vi "Read dotNET Product Definitions.vi"(8 "error in (no error)":errorcluster, 10 "Product Definitions":refnum<k24>[](array[refnum]), 11 "Bundle Builder in":refnum<class "Bundle Builder.lvclass">) -> (0 "error out":errorcluster, 3 "Bundle Builder out":refnum<class "Bundle Builder.lvclass">)   [LabVIEW 2020, in "Bundle Builder.lvclass"]
uses:
  Bundle Builder.lvclass
  C:/Users/chihong/Documents/Repos/StsCustomBundleBuilder/Code/StsCustomBundleBuilderLib/StsCustomBundleBuilderLib/bin/Debug/StsCustomBundleBuilderLib.dll
  StsCustomBundleBuilderLib/StsCustomBundleBuilderLib/bin/Debug/StsCustomBundleBuilderLib.dll
  Bundle Builder.lvclass/Bundle Builder.ctl
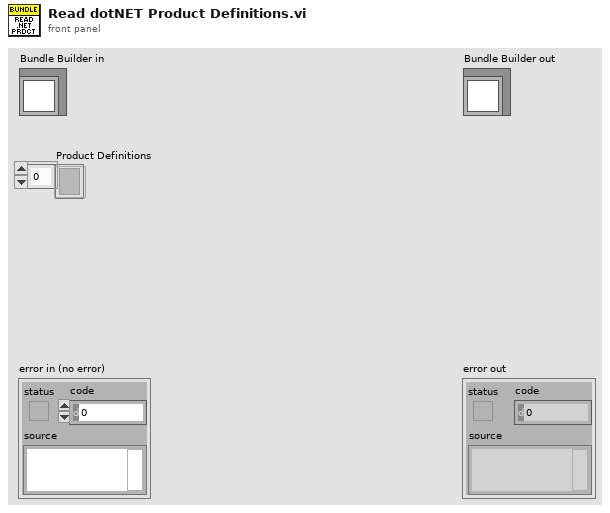
[diagram p1: front panel]
types:
  T1 = cluster{"Display Name":string, "Type":enum16{"NI Installer", "Custom Installer"}, "Install Commands":cluster{"Path":string, "Parameters":string, "Successful Exit Codes":string, "Log Command":cluster{"Flag":string, "File Name":string}}[], "Uninstall Commands":cluster{"Path":string, "Parameters":string, "Successful Exit Codes":string, "Log Command":cluster{"Flag":string, "File Name":string}}[]}
  T2 = cluster{"Path":string, "Parameters":string, "Successful Exit Codes":string, "Log Command":cluster{"Flag":string, "File Name":string}}
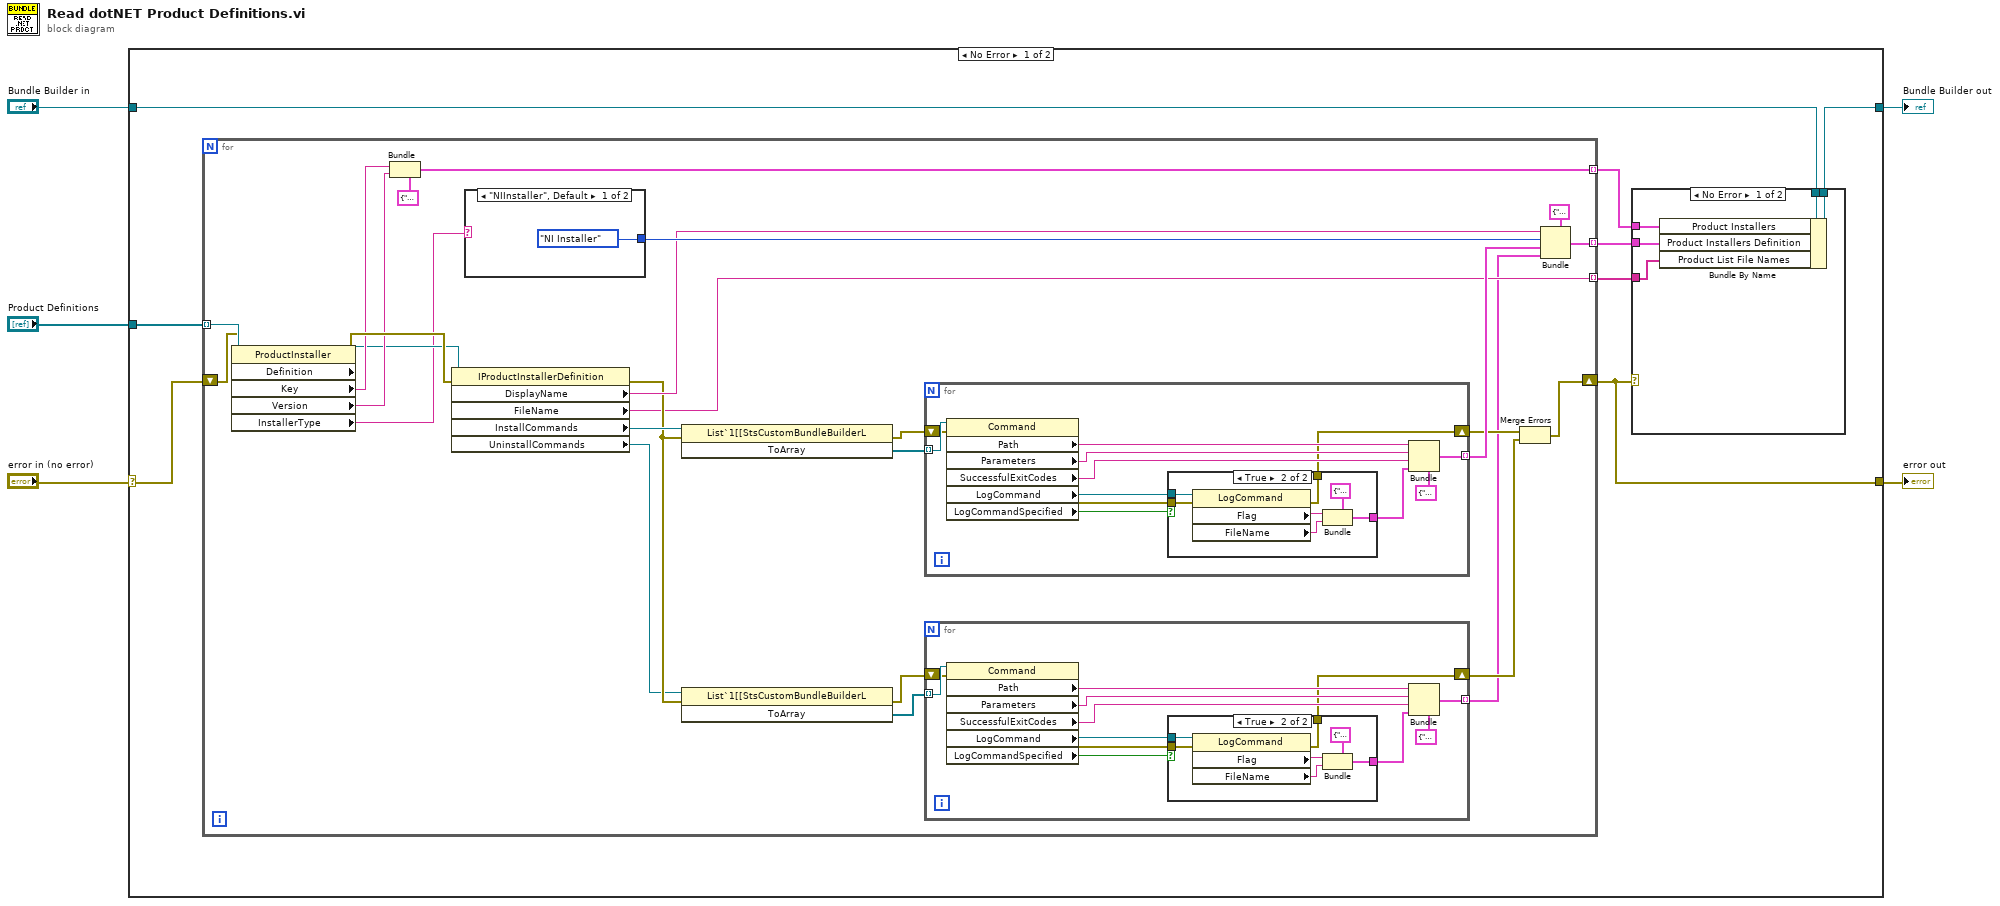
[diagram p0: block diagram]
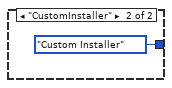
[diagram p5: hidden frame]
diagram:
  n1 = case shown="No Error" "error in (no error)" {
    selector: "error in (no error)" -> [w11 w89]
    tunnel: [w7 w89] -> w4
    tunnel: [w10 w88] -> w2
    tunnel: "Bundle Builder in" -> [w13 w88]
    tunnel: "Product Definitions" -> [w12 _]
    frame No Error {
      n2 = for {
        tunnel: w12 -> [w45] mode=indexing
        shift-right: [w27] -> w7
        shift-left: w11 -> [w44]
        tunnel: [w26] -> w9 mode=indexing
        tunnel: [w25] -> w8 mode=indexing
        tunnel: [w24] -> w6 mode=indexing
        n3 = property class="ProductInstaller"(reference=w45, error in=w44) -> (error out=w43:errorcluster, "Definition"=w38:refnum<k24>, "Key"=w41:string, "Version"=w40:string, "InstallerType"=w37:string)  [unwired: 1 out]
        n4 = Bundle(cluster=cluster{"Key":string, "Version":string} {"Key"="", "Version"=""} ("Product Installer"), "Key"=w41, "Version"=w40) -> (w25:cluster{"Key":string, "Version":string})
        n5 = property class="IProductInstallerDefinition"(reference=w38, error in=w43) -> (error out=w33:errorcluster, "DisplayName"=w35:string, "FileName"=w24:string, "InstallCommands"=w34:refnum<k24>, "UninstallCommands"=w32:refnum<k24>)  [unwired: 1 out]
        n6 = case shown="\"NIInstaller\", Default" w37 {
          tunnel: [enum16{"NI Installer", "Custom Installer"}."NI Installer" ("Type") enum16{"NI Installer", "Custom Installer"}."Custom Installer" ("Type")] -> w36
          frame "NIInstaller", Default {
          }
          frame "CustomInstaller" {
          }
        }
        n7 = invoke class="List`1[[StsCustomBundleBuilderL" method="ToArray"(reference=w34, error in=w33) -> (error out=w30:errorcluster, "ToArray"=w31:refnum<k24>[])  [unwired: 1 in, 1 out]
        n8 = invoke class="List`1[[StsCustomBundleBuilderL" method="ToArray"(reference=w32, error in=w33) -> (error out=w22:errorcluster, "ToArray"=w23:refnum<k24>[])  [unwired: 1 in, 1 out]
        n9 = for {
          tunnel: w31 -> [w77] mode=indexing
          tunnel: [w68] -> w29 mode=indexing
          shift-right: [w67] -> w28
          shift-left: w30 -> [w71]
          n10 = property class="Command"(reference=w77, error in=w71) -> (error out=w72:errorcluster, "Path"=w75:string, "Parameters"=w74:string, "SuccessfulExitCodes"=w70:string, "LogCommand"=w73:refnum<k24>, "LogCommandSpecified"=w66:bool)  [unwired: 1 out]
          n11 = case shown="True" w66 {
            tunnel: w73 -> [_ w85]
            tunnel: w72 -> [w78 w84]
            tunnel: [_ w82] -> w69
            tunnel: [w78 w79] -> w67
            frame False {
            }
            frame True {
              n12 = property class="LogCommand"(reference=w85, error in=w84) -> (error out=w79:errorcluster, "Flag"=w81:string, "FileName"=w80:string)  [unwired: 1 out]
              n13 = Bundle(cluster=cluster{"Flag":string, "File Name":string} {"Flag"="", "File Name"=""} ("Log Command"), "Flag"=w81, "File Name"=w80) -> (w82:cluster{"Flag":string, "File Name":string})
            }
          }
          n14 = Bundle(cluster=T2 {"Path"="", "Parameters"="", "Successful Exit Codes"="", "Log Command"={"Flag"="", "File Name"=""}} ("Product Installer"), "Path"=w75, "Parameters"=w74, "Successful Exit Codes"=w70, "Log Command"=w69) -> (w68:T2)
        }
        n15 = for {
          tunnel: w23 -> [w57] mode=indexing
          tunnel: [w48] -> w20 mode=indexing
          shift-right: [w47] -> w21
          shift-left: w22 -> [w51]
          n16 = property class="Command"(reference=w57, error in=w51) -> (error out=w52:errorcluster, "Path"=w55:string, "Parameters"=w54:string, "SuccessfulExitCodes"=w50:string, "LogCommand"=w53:refnum<k24>, "LogCommandSpecified"=w46:bool)  [unwired: 1 out]
          n17 = case shown="True" w46 {
            tunnel: w53 -> [_ w65]
            tunnel: w52 -> [w58 w64]
            tunnel: [_ w62] -> w49
            tunnel: [w58 w59] -> w47
            frame False {
            }
            frame True {
              n18 = property class="LogCommand"(reference=w65, error in=w64) -> (error out=w59:errorcluster, "Flag"=w61:string, "FileName"=w60:string)  [unwired: 1 out]
              n19 = Bundle(cluster=cluster{"Flag":string, "File Name":string} {"Flag"="", "File Name"=""} ("Log Command"), "Flag"=w61, "File Name"=w60) -> (w62:cluster{"Flag":string, "File Name":string})
            }
          }
          n20 = Bundle(cluster=T2 {"Path"="", "Parameters"="", "Successful Exit Codes"="", "Log Command"={"Flag"="", "File Name"=""}} ("Product Installer"), "Path"=w55, "Parameters"=w54, "Successful Exit Codes"=w50, "Log Command"=w49) -> (w48:T2)
        }
        n21 = Merge Errors(w28, w21) -> (w27:errorcluster)
        n22 = Bundle(cluster=T1 {"Display Name"="", "Type"=enum."NI Installer", "Install Commands"=[], "Uninstall Commands"=[]} ("Product Installer"), "Display Name"=w35, "Type"=w36, "Install Commands"=w29, "Uninstall Commands"=w20) -> (w26:T1)
      }
      n23 = case shown="No Error" w7 {
        tunnel: w13 -> [w18 w19]
        tunnel: [w17 w19] -> w10
        tunnel: w9 -> [w16 _]
        tunnel: w8 -> [w15 _]
        tunnel: w6 -> [w14 _]
        frame No Error {
          n24 = Bundle By Name(cluster=w18, "Product Installers"=w15, "Product Installers Definition"=w16, "Product List File Names"=w14) -> (w17:refnum<class "Bundle Builder.lvclass">)
        }
        frame Error {
        }
      }
    }
    frame Error {
    }
  }
  "error out" <- w4
  "Bundle Builder out" <- w2
